vi "Close FP.vi"(8 "Error In":errorcluster, 11 "VI Ref":refnum<vi>) -> (0 "Error Out":errorcluster)   [LabVIEW 2019, in "LMH-Toolbox.lvlib"]
doc: "Close the VI front panel. If the user is holding shift while the FP would close it is left open (for debugging)."
uses:
  <vilib>/MakerHub/Toolbox/LMH-Toolbox.lvlib
  <vilib>/Utility/inputDevices.llb/closeKeyboard.vi
  <vilib>/Utility/inputDevices.llb/keyboardAcquire.vi
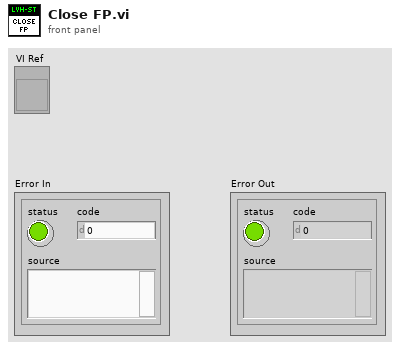
[diagram p1: front panel]
types:
  T1 = enum16{"0", "1", "2", "3", "4", "5", "6", "7", "8", "9", "A", "B", "C", "D", "E", "F", "G", "H", "I", "J", "K", "L", "M", "N", "O", "P", "Q", "R", "S", "T", "U", "V", "W", "X", "Y", "Z", "F1", "F2", "F3", "F4", "F5", "F6", "F7", "F8", "F9", "F10", "F11", "F12", "F13", "F14", "F15", "ADD", "BACK", "BACKSLASH", "CAPITAL", "COMMA", "DECIMAL", "DELETE", "DIVIDE", "DOWN", "END", "EQUALS", "ESCAPE", "GRAVE (`)", "HOME", "INSERT", "LBRACKET", "LCONTROL", "LEFT", "L ALT", "LSHIFT", "LWIN", "MINUS", "MULTIPLY", "NEXT", "NUMLOCK", "NUMPAD_0", "NUMPAD_1", "NUMPAD_2", "NUMPAD_3", "NUMPAD_4", "NUMPAD_5", "NUMPAD_6", "NUMPAD_7", "NUMPAD_8", "NUMPAD_9", "PAUSE", "PERIOD", "PRIOR (PG UP)", "RBRACKET", "RCONTROL", "RETURN", "RIGHT", "R ALT", "RSHIFT", "RWIN", "SCROLL", "SEMICOLON", "SLASH", "SPACE", "SUBTRACT", "TAB", "UP", "ENTER (num pad)", "' (quote)"}[]
  T2 = enum16{"0", "1", "2", "3", "4", "5", "6", "7", "8", "9", "A", "B", "C", "D", "E", "F", "G", "H", "I", "J", "K", "L", "M", "N", "O", "P", "Q", "R", "S", "T", "U", "V", "W", "X", "Y", "Z", "F1", "F2", "F3", "F4", "F5", "F6", "F7", "F8", "F9", "F10", "F11", "F12", "F13", "F14", "F15", "ADD", "BACK", "BACKSLASH", "CAPITAL", "COMMA", "DECIMAL", "DELETE", "DIVIDE", "DOWN", "END", "EQUALS", "ESCAPE", "GRAVE (`)", "HOME", "INSERT", "LBRACKET", "LCONTROL", "LEFT", "L ALT", "LSHIFT", "LWIN", "MINUS", "MULTIPLY", "NEXT", "NUMLOCK", "NUMPAD_0", "NUMPAD_1", "NUMPAD_2", "NUMPAD_3", "NUMPAD_4", "NUMPAD_5", "NUMPAD_6", "NUMPAD_7", "NUMPAD_8", "NUMPAD_9", "PAUSE", "PERIOD", "PRIOR (PG UP)", "RBRACKET", "RCONTROL", "RETURN", "RIGHT", "R ALT", "RSHIFT", "RWIN", "SCROLL", "SEMICOLON", "SLASH", "SPACE", "SUBTRACT", "TAB", "UP", "ENTER (num pad)", "' (quote)"}
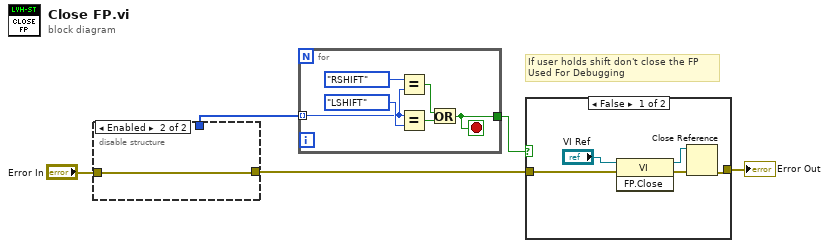
[diagram p0: block diagram]
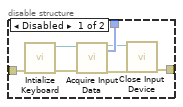
[diagram p2: hidden frame]
diagram:
  # "If user holds shift don't close the FP\nUsed For Debugging"
  n1 = disable-structure shown="Enabled" {
    disable-tunnel: [w12 _] -> w4
    disable-tunnel: [w7 w13] -> w3
    disable-tunnel: "Error In" -> [w6 w13]
    frame Disabled {
      n2 = call <vilib>:"Intialize Keyboard.vi"("error in (no error)"=w6) -> ("error out"=w8:errorcluster, "device ID"=w9:refnum<k1>)  [unwired: 9 in]
      n3 = call-poly <vilib>:"Acquire Input Data.vi"("device ID"=w9, "error in (no error)"=w8) -> ("device ID"=w11:refnum<k1>, "keys pressed"=w12:T1, "error out"=w10:errorcluster)  [unwired: 15 in]
      n4 = call-poly <vilib>:"Close Input Device.vi"("error in (no error)"=w10, "device ID"=w11) -> ("error out"=w7:errorcluster)  [unwired: 8 in]
    }
    frame Enabled {
    }
  }
  n5 = for {
    tunnel: w4 -> [w16] mode=indexing
    tunnel: [w14] -> w2
    stop <- w14 stop-if-true
    n6 = Equal?(x=T2."RSHIFT", y=w16) -> (x = y?=w18:bool)
    n7 = Equal?(x=w16, y=T2."LSHIFT" ("x")) -> (x = y?=w15:bool)
    n8 = Or(x=w18, y=w15) -> (x .or. y?=w14:bool)
  }
  n9 = case shown="False" w2 {
    tunnel: [w24 w25] -> w5
    tunnel: w3 -> [w21 w25]
    frame False {
      n10 = invoke class="VI" method="FP.Close"(reference="VI Ref", error in=w21) -> (reference out=w22:refnum<vi>, error out=w23:errorcluster)  [unwired: 1 in, 1 out]
      n11 = Close Reference(reference=w22, error in (no error)=w23) -> (error out=w24:errorcluster)
    }
    frame True {
    }
  }
  "Error Out" <- w5
